vi "Ultrasonic Transducers.vi"() -> ()   [LabVIEW 2014]
panel:
  out "x >= y?":bool
  in  "Tab Control":T1(tab)
  out "?":bool
  out "?":bool
  out "?":bool
  out "?":bool
  out "?":bool
  out "?":bool
  out "?":bool
  out "?":bool
  out "?":bool
  out "?":bool
  out "?":bool
  out "?":bool
  out "?":bool
  out "?":bool
  out "?":dbl(slide) scale=0.0..800.0
  out "?":dbl format="%#_4g"
  out "?":dbl format="%#_4g"
  out "Level (in mm) Vs Transmitter Current (mA)":cluster{"Y":dbl[], "Y":dbl[]}[](graph)
  out "1 2":string[][](table)
  out "?":dbl(slide) scale=0.0..800.0
  out "?":dbl(slide) scale=0.0..800.0
  out "1":string[][](table)
  in  "?":dbl(slide)=29.292929292929294 scale=0.0..100.0
  out "Level (in mm) Vs Transmitter Current (mA)":cluster{"Y":dbl[], "Y":dbl[]}[](graph)
  out "?":dbl(slide) scale=0.0..800.0
  out "?":dbl format="%#_4g"
  out "?":dbl format="%#_4g"
  # "Manipal Institute of Technology  \n        Dept of Instrumentation and Control Engineering\n                                 V Sem (Instrumentation Lab)"
  # "VIRTUAL LABS"
  # "VIRTUAL LABS"
  # "Measurement of Level Using Ultrasonic Transducer\n \nAim:\nTo measure the liquid level in the process tank using Ultrasonic Transducer.\n Apparatus required:\n1\tVLMT-04 Unit.\n2\tPatch Chord.\n3\tDMM\n\n\nInstructions:\n1.\tSwitch ON the Trainer. \n2.\tThe Pump inlet valve (HV1) should be fully open and the process tank outlet valve HV2 should be fully closed. \n3.\tConnect the multimeter across (4-20) mA.\n4.\tVary the pump speed using variable speed knob, set the level at 0mm. \n5.\tNote the transmitter output in (4-20) mA terminals.\n6.\tGradually increase the water level by using variable speed knob and note down the water level and transmitter output.\n7.\tPlot the Graph between level (mm) and transmitter output (mA) along x-axis and y-axis respectively."
  # "EXPERIMENT NO.1"
  # "Level in (mm)"
  # "Transmitter o/p (mA)"
  # "Study Of Float Type Level Transmitter\n\nAim:\n\nTo measure the liquid level in the process tank using float type level transmitter.\nApparatus required:\n1\tVLMT-05 Unit.\n2\tPatch Chord.\n3\tDMM\n\nInstructions:\n\n1.\tSwitch ON the Trainer.\n2.\tThe Pump inlet valve (HV1) should be fully open and the process tank outlet valve HV2 should be fully closed.\n3.\tConnect the multimeter across (L1 and L2) in (DC - mA) mode.\n4.\tVary the pump speed using variable speed knob, set the level at 0mm.\n5.\tNote the transmitter output in Ll, L2 terminals.\n6.\tGradually increase the water level by using variable speed knob and note down the water level and transmitter output.\n7.\tPlot the graph between level (mm) and transmitter output (mA) along x and y-axis respectively."
  # "Level in (mm)"
  # "Animation Speed"
  # "Transmitter o/p (mA)"
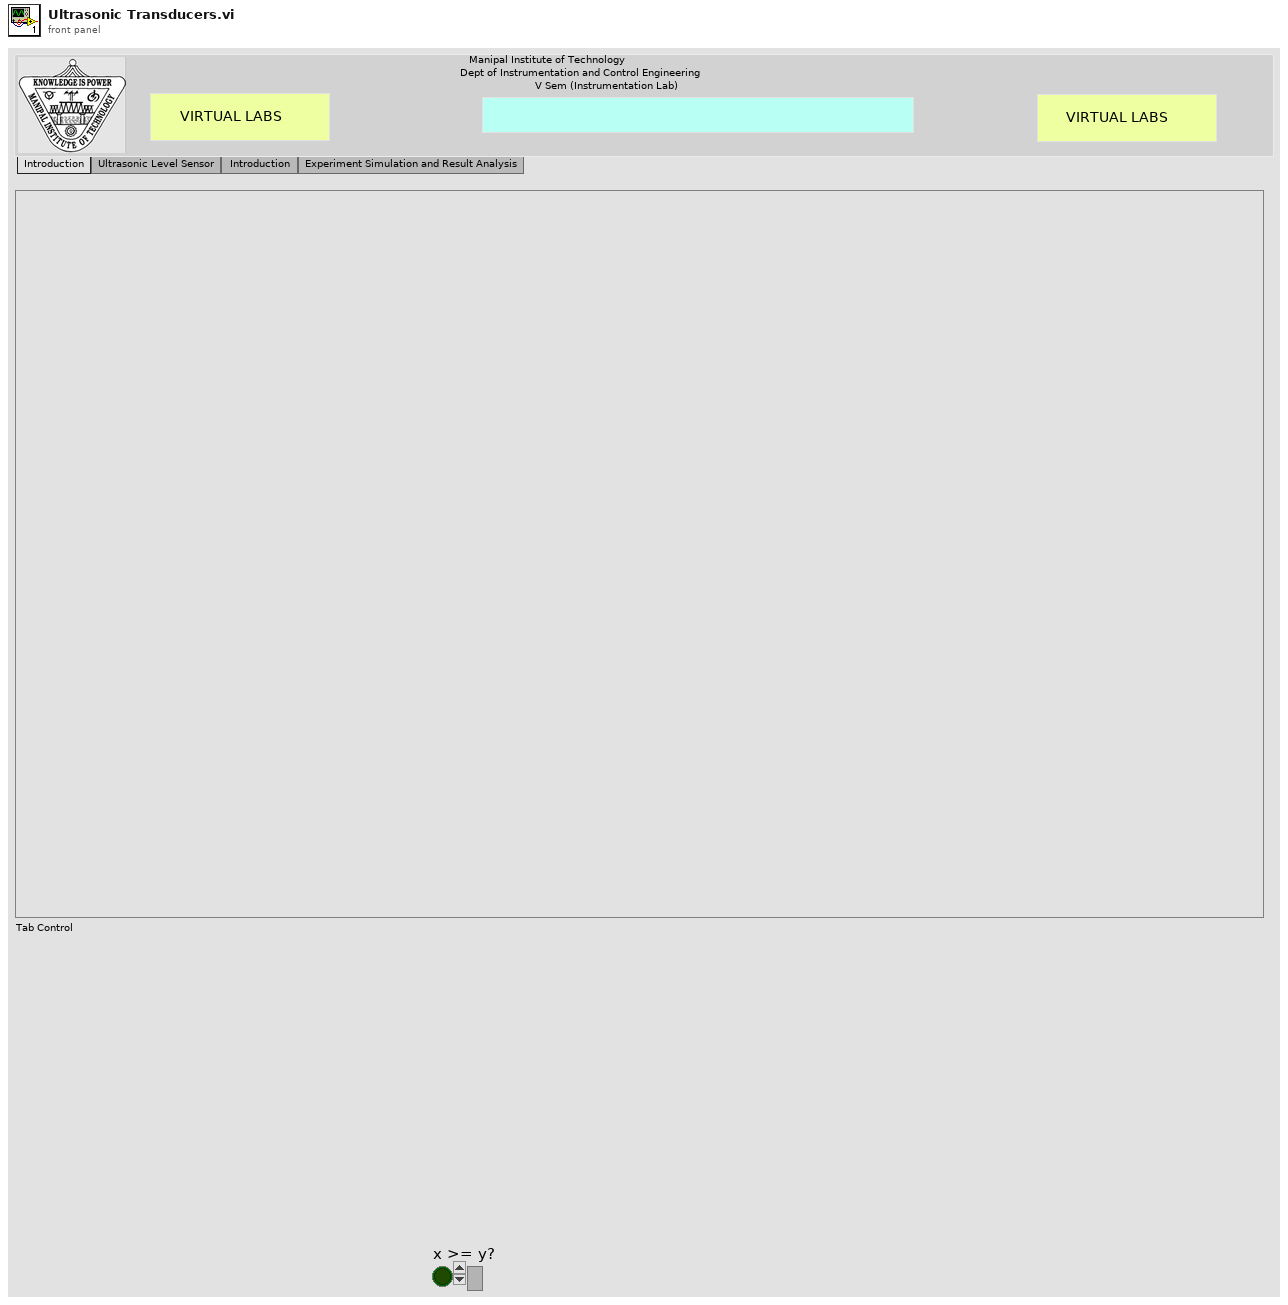
[diagram p1: front panel]
types:
  T1 = enum32{"Introduction", "Ultrasonic Level Sensor", "Introduction ", "Experiment Simulation and Result Analysis"}
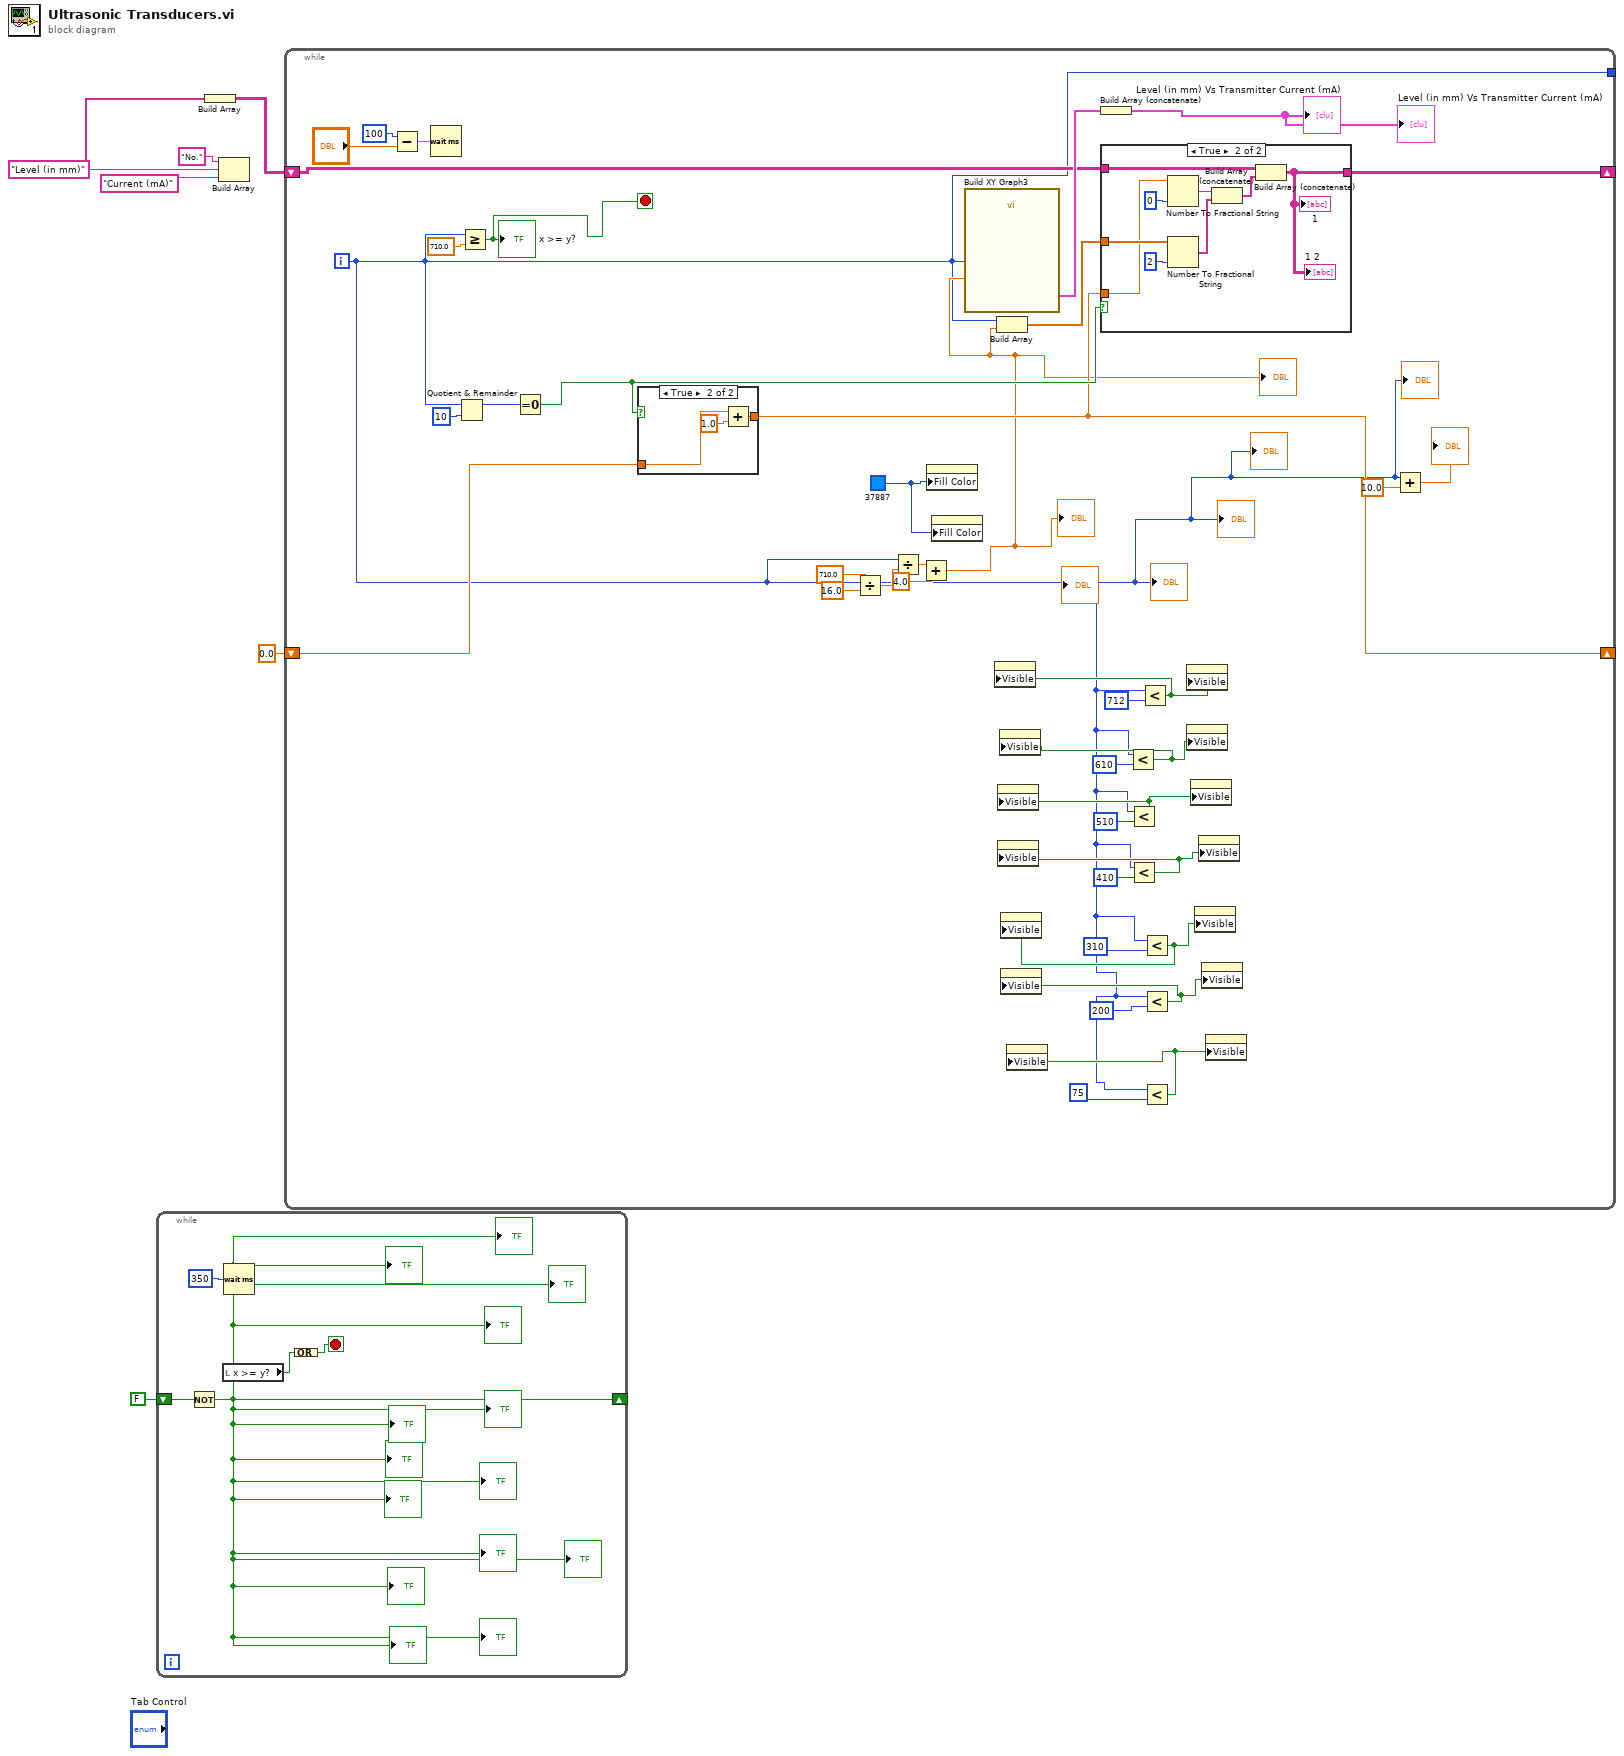
[diagram p0: block diagram]
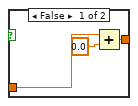
[diagram p2: hidden frame]
diagram:
  n1 = while {
    shift-right: [w8] -> _
    shift-left: FALSE -> [w12]
    stop <- w9 stop-if-true
    n2 = Not(x=w12) -> (.not. x?=w8:bool)
    "?" <- w8
    "?" <- w8
    "?" <- w8
    "?" <- w8
    "?" <- w8
    "?" <- w8
    "?" <- w8
    "?" <- w8
    "?" <- w8
    "?" <- w8
    "?" <- w8
    "?" <- w8
    "?" <- w8
    "?" <- w8
    n3 = local read "x >= y?"() -> (w10:bool)
    n4 = Wait (ms)(milliseconds to wait=u32 350) -> ()  [unwired: 1 out]
    n5 = Compound Arithmetic op=OR(w10) -> (w9:bool)
  }
  n6 = Build Array("No." ("element"), "Level (in mm)" ("element"), "Current (mA)") -> (w4:string[])
  n7 = Build Array(w4) -> (w3:string[][])
  n8 = while {
    tunnel: [w13] -> _
    shift-right: [w45] -> _
    shift-left: w3 -> [w46]
    shift-right: [w19] -> _
    shift-left: 0.0 -> [w42]
    i -> [w13]
    stop <- w39 stop-if-true
    w20 = u32 37887
    n9 = Subtract(x=u32 100 ("milliseconds to wait"), y="?") -> (x-y=w48:dbl)
    n10 = Wait (ms)(milliseconds to wait=w48) -> ()  [unwired: 1 out]
    n11 = Quotient & Remainder(x=w13, y=10) -> (x-y*floor(x/y)=w44:i32)  [unwired: 1 out]
    n12 = Greater Or Equal?(x=w13, y=710.0) -> (x >= y?=w39:bool)
    "x >= y?" <- w39
    n13 = Equal To 0?(x=w44) -> (x = 0?=w40:bool)
    n14 = case shown="True" w40 {
      tunnel: w42 -> [w53 w57]
      tunnel: [w52 w56] -> w19
      frame False {
        n15 = Add(x=w53, y=0.0) -> (x+y=w52:dbl)
      }
      frame True {
        n16 = Add(x=w57, y=1.0) -> (x+y=w56:dbl)
      }
    }
    n17 = Divide(x=710.0, y=16.0) -> (x/y=w36:dbl)
    n18 = Divide(x=w13, y=w36) -> (x/y=w35:dbl)
    n19 = Add(x=w35, y=4.0) -> (x+y=w16:dbl)
    "?" <- w16
    "?" <- w16
    n20 = property class="Slide (strict)"("Fill Color"=w20) -> ()  [unwired: 2 in, 2 out]
    n21 = property class="Slide (strict)"("Fill Color"=w20) -> ()  [unwired: 2 in, 2 out]
    n22 = call "Build XY Graph3"("Y Input"=w16, "X Input"=w13) -> ("XY Graph"=w50:cluster{"Y":dbl[], "Y":dbl[]}[])  [unwired: 3 in, 6 out]
    n23 = Build Array(w13, w16) -> (w41:dbl[])
    n24 = Build Array (concatenate)(w50) -> (→"Level (in mm) Vs Transmitter Current (mA)" →"Level (in mm) Vs Transmitter Current (mA)":cluster{"Y":dbl[], "Y":dbl[]}[])
    n25 = case shown="True" w40 {
      tunnel: w41 -> [_ w67]
      tunnel: w46 -> [w58 w60]
      tunnel: [w58 w59] -> w45
      tunnel: w19 -> [_ w65]
      frame False {
      }
      frame True {
        n26 = Number To Fractional String(number=w65, precision (6)=i16 0) -> (F-format string=w63:string)  [unwired: 2 in]
        n27 = Number To Fractional String(number=w67, precision (6)=i16 2) -> (F-format string=w62:string[])  [unwired: 2 in]
        n28 = Build Array (concatenate)(w63, w62) -> (w61:string[])
        n29 = Build Array (concatenate)(w60, w61) -> (w59:string[][])
        "1" <- w59
        "1 2" <- w59
      }
    }
    n30 = Less?(x=w13, y=610) -> (x < y?=w29:bool)
    n31 = property class="Bool (strict)"("Visible"=w29) -> ()  [unwired: 2 in, 2 out]
    n32 = Less?(x=w13, y=510) -> (x < y?=w28:bool)
    n33 = property class="Bool (strict)"("Visible"=w28) -> ()  [unwired: 2 in, 2 out]
    n34 = Less?(x=w13, y=410) -> (x < y?=w27:bool)
    n35 = property class="Bool (strict)"("Visible"=w27) -> ()  [unwired: 2 in, 2 out]
    n36 = Less?(x=w13, y=712) -> (x < y?=w14:bool)
    n37 = property class="Bool (strict)"("Visible"=w14) -> ()  [unwired: 2 in, 2 out]
    n38 = Less?(x=w13, y=310) -> (x < y?=w26:bool)
    n39 = property class="Bool (strict)"("Visible"=w26) -> ()  [unwired: 2 in, 2 out]
    n40 = Less?(x=w13, y=200) -> (x < y?=w23:bool)
    n41 = property class="Bool (strict)"("Visible"=w23) -> ()  [unwired: 2 in, 2 out]
    n42 = Less?(x=w13, y=75) -> (x < y?=w22:bool)
    n43 = property class="Bool (strict)"("Visible"=w22) -> ()  [unwired: 2 in, 2 out]
    n44 = property class="Bool (strict)"("Visible"=w14) -> ()  [unwired: 2 in, 2 out]
    n45 = property class="Bool (strict)"("Visible"=w29) -> ()  [unwired: 2 in, 2 out]
    n46 = property class="Bool (strict)"("Visible"=w28) -> ()  [unwired: 2 in, 2 out]
    n47 = property class="Bool (strict)"("Visible"=w26) -> ()  [unwired: 2 in, 2 out]
    n48 = property class="Bool (strict)"("Visible"=w27) -> ()  [unwired: 2 in, 2 out]
    n49 = property class="Bool (strict)"("Visible"=w23) -> ()  [unwired: 2 in, 2 out]
    n50 = property class="Bool (strict)"("Visible"=w22) -> ()  [unwired: 2 in, 2 out]
    n51 = Add(x=w13, y=10.0) -> (x+y=→"?":dbl)
    "?" <- w13
    "?" <- w13
    "?" <- w13
    "?" <- w13
    "?" <- w13
  }
